vi "Swerve Setpoints FGV.vi"(1 "New Setpoint":dbl format="%#_13g", 2 "Swerve Number":enum16{"1", "2", "3", "4"}(ring), 3 "Action":enum16{"Set", "Get"}(ring)=enum."Get") -> (0 "Setpoint":dbl)   [LabVIEW 2017, in "Huskie Swerve.lvlib"]
uses:
  Huskie Swerve.lvlib
panel:
  out "x-y*floor(x/y)":dbl[](array[numeric])
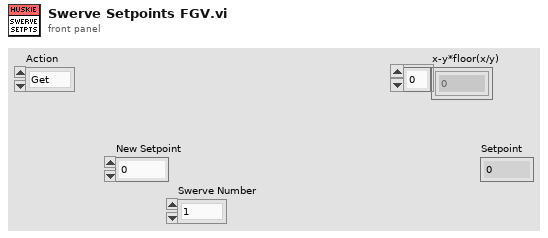
[diagram p1: front panel]
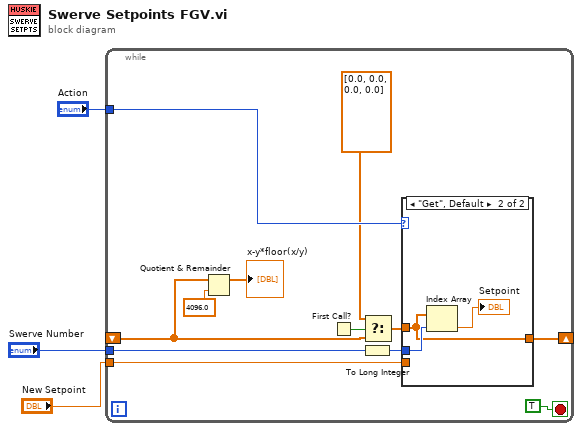
[diagram p0: block diagram]
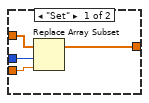
[diagram p2: hidden frame]
diagram:
  n1 = while {
    shift-right: [w10] -> _
    shift-left: _ -> [w6]
    tunnel: "New Setpoint" -> [w11]
    tunnel: "Action" -> [w14]
    tunnel: "Swerve Number" -> [w13]
    stop <- TRUE stop-if-true
    n2 = Quotient & Remainder(x=w6, y=4096.0) -> (x-y*floor(x/y)=→"x-y*floor(x/y)":dbl[])  [unwired: 1 out]
    n3 = First Call?() -> (First Call?: T/F=w9:bool)
    n4 = To Long Integer(number=w13) -> (32bit integer=w12:i32)
    n5 = Select(t=dbl[] [0.0, 0.0, 0.0, 0.0], s=w9, f=w6) -> (s? t:f=w7:dbl[])
    n6 = case shown="\"Get\", Default" w14 {
      tunnel: w7 -> [w19 w20]
      tunnel: w12 -> [w18 w22]
      tunnel: w11 -> [w17 _]
      tunnel: [w16 w20] -> w10
      frame "Set" {
        n7 = Replace Array Subset(array=w19, new element=w17, index=w18) -> (w16:dbl[])
      }
      frame "Get", Default {
        n8 = Index Array(array=w20, index=w22) -> (element=→"Setpoint":dbl)
      }
    }
  }
